vi "Get Unitless Values.vi"(8 "error in (no error)":errorcluster, 11 "Analyze Results Beam Deviation in":refnum<class "Analyze Results Beam Deviation.lvclass">) -> (0 "error out":errorcluster, 2 "UnitLess Values":T1[](array[typedef]), 3 "Analyze Results Beam Deviation out":refnum<class "Analyze Results Beam Deviation.lvclass">)   [LabVIEW 2020, in "Analyze Results Beam Deviation.lvclass"]
uses:
  Analyze Results Beam Deviation.lvclass
  Results Base/UnitLessValue.ctl
  Analyze Results Beam Deviation.lvclass/Analyze Results Beam Deviation.ctl
  Results Base/Analyze Results Base.lvclass
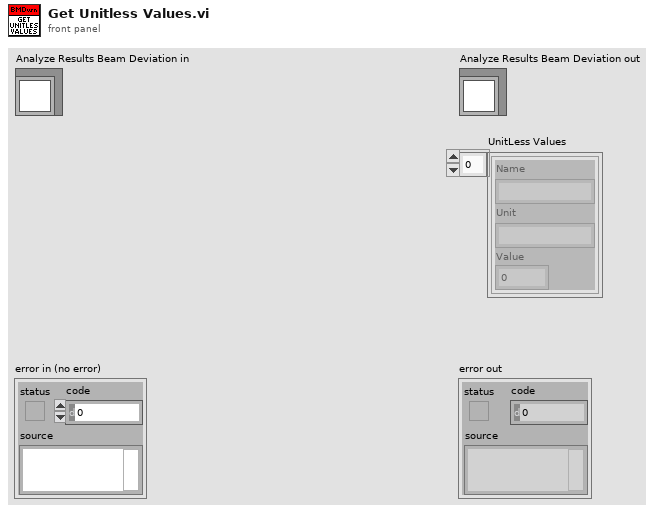
[diagram p1: front panel]
types:
  T1 = typedef "Analyze Results Base.lvclass/UnitLessValue.ctl" = cluster{"Name":string, "Unit":string, "Value":dbl}
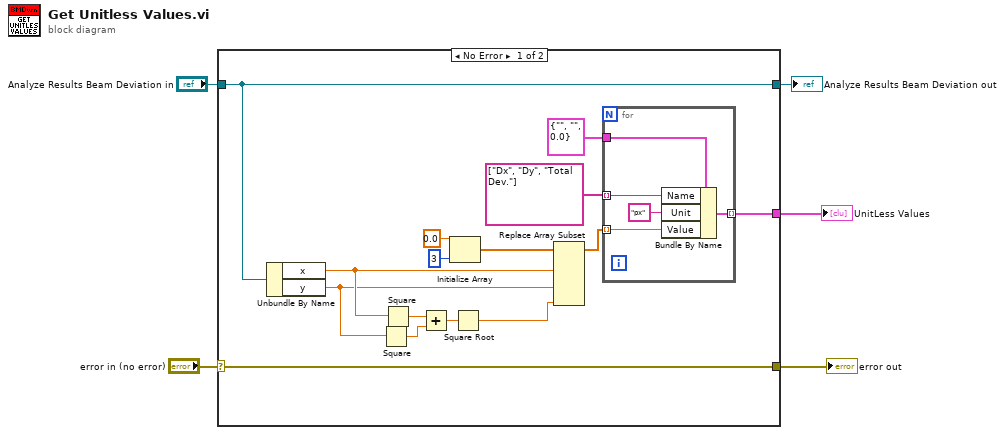
[diagram p0: block diagram]
diagram:
  n1 = case shown="No Error" "error in (no error)" {
    selector: "error in (no error)" -> [w6 w26]
    tunnel: "Analyze Results Beam Deviation in" -> [w7 w27]
    tunnel: [w8 _] -> w4
    tunnel: [w7 w27] -> w3
    tunnel: [w6 w26] -> w2
    frame No Error {
      n2 = Unbundle By Name(w7) -> ("x"=w14:sgl, "y"=w13:sgl)
      n3 = Square(x=w13) -> (x^2=w18:sgl)
      n4 = Square(x=w14) -> (x^2=w19:sgl)
      n5 = Add(x=w19, y=w18) -> (x+y=w20:sgl)
      n6 = Initialize Array(sgl 0.0 ("element"), 3 ("dimension size")) -> (w16:sgl[])
      n7 = Square Root(x=w20) -> (sqrt(x)=w12:sgl)
      n8 = Replace Array Subset(array=w16, new element #1=w14, new element #2=w13, new element #3=w12) -> (w11:sgl[])  [unwired: 3 in]
      n9 = for {
        tunnel: w11 -> [w21] mode=indexing
        tunnel: string[] ["Dx", "Dy", "Total Dev."] -> [w23] mode=indexing
        tunnel: T1 {"Name"="", "Unit"="", "Value"=0.0} ("UnitLessValue") -> [w25]
        tunnel: [w24] -> w8 mode=indexing
        n10 = Bundle By Name(cluster=w25, "Name"=w23, "Unit"="px", "Value"=w21) -> (w24:T1)
      }
    }
    frame Error {
    }
  }
  "error out" <- w2
  "Analyze Results Beam Deviation out" <- w3
  "UnitLess Values" <- w4
